vi "update pid.vi"(8 "error in (no error)":errorcluster, 9 "PID gains":T1, 10 "config path":path, 11 "Dynamic-System in":refnum<class "Dynamic-System.lvclass">) -> (0 "error out":errorcluster, 3 "Dynamic-System out":refnum<class "Dynamic-System.lvclass">)   [LabVIEW 2025, in "Dynamic-System.lvclass"]
uses:
  Dynamic-System.lvclass
  66534c67-6d14-48c8-9a05-17613b7a0829.vi
  <vilib>/JDP Science/JSONtext/JSON text to Variant.vi
  <vilib>/JDP Science/JSONtext/LVClass Serializer/JSONtext LVClass Serializer.lvclass
  Dynamic-System.lvclass/Dynamic-System.ctl
  <vilib>/JDP Science/JSONtext/JSONtext.lvlib
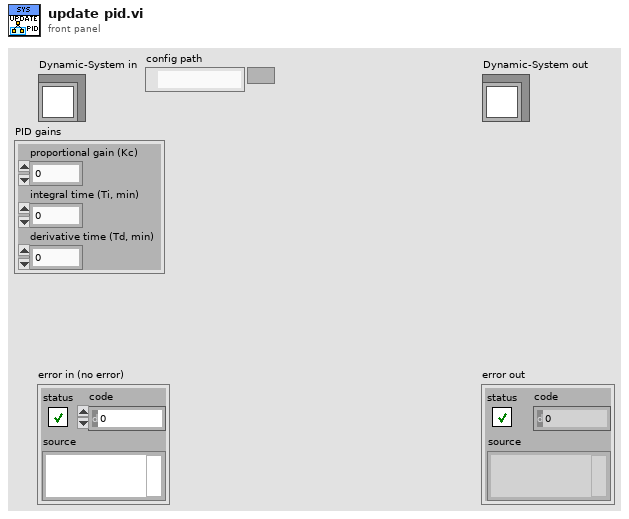
[diagram p1: front panel]
types:
  T1 = cluster{"proportional gain (Kc)":dbl, "integral time (Ti, min)":dbl, "derivative time (Td, min)":dbl}
  T2 = enum16{"open", "replace", "create", "open or create", "replace or create", "replace or create with confirmation"}
  T3 = cluster{"State_Equations":string[], "State_Variables":string[], "Initial_Conditions":dbl[], "Step_size":dbl, "Data":dbl[][], "Parameters":cluster{"Param1":dbl, "Param2":dbl}, "T_f":dbl, "Input":string, "PID_gains":cluster{"P":dbl, "I":dbl, "D":dbl}}
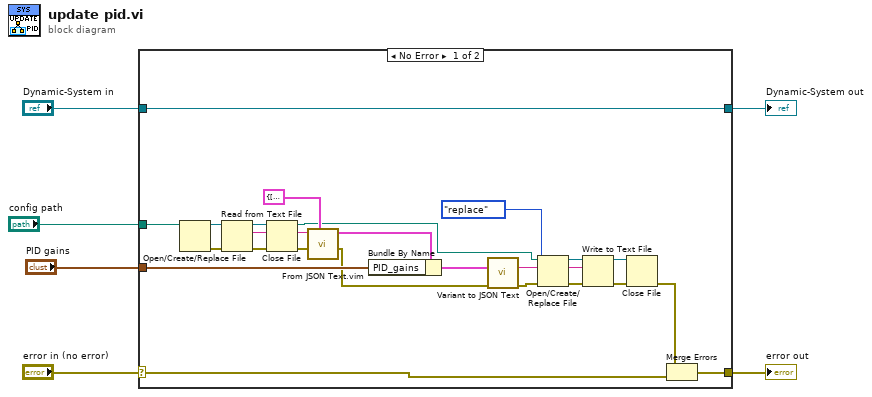
[diagram p0: block diagram]
diagram:
  n1 = case shown="No Error" "error in (no error)" {
    selector: "error in (no error)" -> [w9 w32]
    tunnel: [w8 w32] -> w5
    tunnel: [w20 w31] -> w3
    tunnel: "Dynamic-System in" -> [w20 w31]
    tunnel: "PID gains" -> [w21 _]
    tunnel: "config path" -> [w18 _]
    frame No Error {
      n2 = Open/Create/Replace File(file path (use dialog)=w18) -> (refnum out=w25:refnum<file>, error out=w24:errorcluster)  [unwired: 5 in, 1 out]
      n3 = Read from Text File(file (use dialog)=w25, error in=w24) -> (refnum out=w12:refnum<file>, text=w26:string, error out=w13:errorcluster)  [unwired: 2 in, 1 out]
      n4 = Close File(refnum=w12, error in=w13) -> (path=w10:path, error out=w11:errorcluster)
      n5 = call "From JSON Text.vim"("Data Type and Default Value"=T3 {"State_Equations"=[], "State_Variables"=[], "Initial_Conditions"=[], "Step_size"=0.0, "Data"=[], "Parameters"={"Param1"=0.0, "Param2"=0.0}, "T_f"=0.0, "Input"="+0", "PID_gains"={"P"=0.0, "I"=0.0, "D"=0.0}}, "error in (no error)"=w11, "JSON"=w26) -> ("error out"=w19:errorcluster, "Data out"=w23:T3)  [unwired: 7 in]
      n6 = Bundle By Name(cluster=w23, "PID_gains"=w21) -> (w22:T3)
      n7 = call <vilib>:"Variant to JSON Text.vi"("error in (no error)"=w19, "Variant"=w22) -> ("error out"=w17:errorcluster, "<JSON>"=w28:string)  [unwired: 7 in, 1 out]
      n8 = Open/Create/Replace File(file path (use dialog)=w10, error in=w17, operation (0:open)=T2."replace") -> (refnum out=w15:refnum<file>, error out=w14:errorcluster)  [unwired: 3 in, 1 out]
      n9 = Write to Text File(file (use dialog)=w15, text=w28, error in=w14) -> (refnum out=w29:refnum<file>, error out=w30:errorcluster)  [unwired: 1 in, 1 out]
      n10 = Close File(refnum=w29, error in=w30) -> (error out=w7:errorcluster)  [unwired: 1 out]
      n11 = Merge Errors(w7, w9) -> (w8:errorcluster)
    }
    frame Error {
    }
  }
  "error out" <- w5
  "Dynamic-System out" <- w3
